vi "_GUID.vi"() -> (3 "uuid":string)   [LabVIEW 2014, in "TagDB(dev).lvlib"]
doc: "Generates a unique identification stringCopyright 2015 National Instruments Corporation\n\nLicensed under the Apache License, Version 2.0 (the \"License\"); you may not use this file except in compliance with the License. You may obtain a copy of the License at http://www.apache.org/licenses/LICENSE-2.0\nUnless required by applicable law or agreed to in writing, software distributed under the License is distributed on an \"AS IS\" BASIS, WITHOUT WARRANTIES OR CONDITIONS OF ANY KIND, either express or implied. See the License for the specific language governing permissions and limitations under the License."
uses:
  TagDB(dev).lvlib
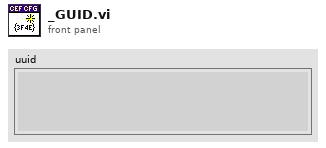
[diagram p1: front panel]
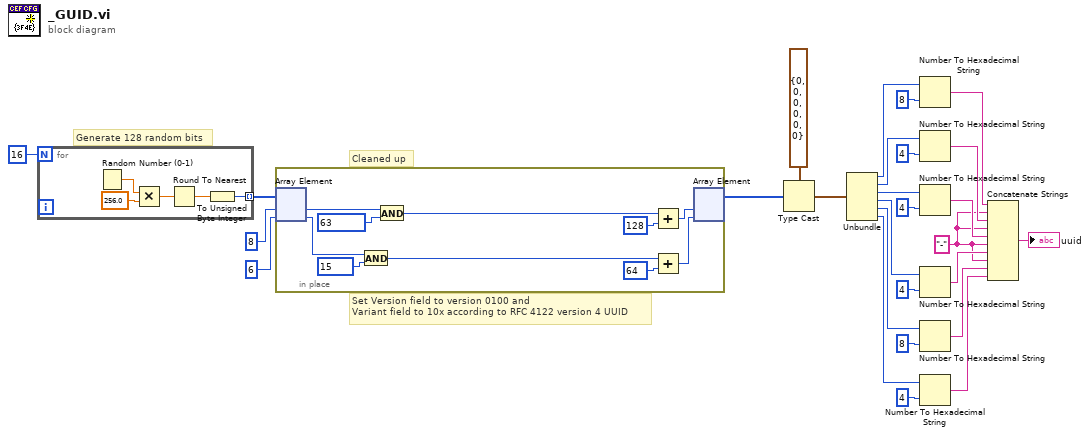
[diagram p0: block diagram]
diagram:
  w11 = "-" ("new element/subarray")
  # "Cleaned up"
  # "Set Version field to version 0100 and \nVariant field to 10x according to RFC 4122 version 4 UUID"
  # "Generate 128 random bits"
  n1 = for {
    N: 16 -> [_]
    tunnel: [w28] -> w26 mode=indexing
    n2 = Random Number (0-1)() -> (number: 0 to 1=w32:dbl)
    n3 = Multiply(x=w32, y=256.0) -> (x*y=w30:dbl)
    n4 = Round To Nearest(number=w30) -> (nearest integer value=w29:dbl)
    n5 = To Unsigned Byte Integer(number=w29) -> (unsigned 8bit integer=w28:u8)
  }
  n6 = in-place {
    n7 = in-place-array #1(w26, 8 ("index"), 6 ("index")) -> (w41:u8, w40:u8)
    n8 = And(x=w40, y=u8 15) -> (x .and. y?=w37:u8)
    n9 = And(x=w41, y=u8 63) -> (x .and. y?=w35:u8)
    n10 = Add(x=w35, y=u8 128) -> (x+y=w34:u8)
    n11 = Add(x=w37, y=u8 64) -> (x+y=w33:u8)
    n12 = in-place-array #1(w34, w33) -> (w2:u8[])  [unwired: 2 out]
  }
  n13 = Type Cast(type=cluster{u32, u16, u16, u16, u32, u16} {0, 0, 0, 0, 0, 0}, x=w2) -> (*(type *) &x=w22:cluster{u32, u16, u16, u16, u32, u16})
  n14 = Unbundle(w22) -> (w8:u32, w7:u16, w6:u16, w5:u16, w4:u32, w3:u16)
  n15 = Number To Hexadecimal String(1:i16 8 ("width (-)"), 2:w8) -> (0:w15:string)
  n16 = Number To Hexadecimal String(1:i16 4 ("width (-)"), 2:w7) -> (0:w14:string)
  n17 = Number To Hexadecimal String(1:i16 4 ("width (-)"), 2:w6) -> (0:w13:string)
  n18 = Number To Hexadecimal String(1:i16 4 ("width (-)"), 2:w5) -> (0:w12:string)
  n19 = Number To Hexadecimal String(1:i16 8 ("width (-)"), 2:w4) -> (0:w10:string)
  n20 = Number To Hexadecimal String(1:i16 4 ("width (-)"), 2:w3) -> (0:w9:string)
  n21 = Concatenate Strings(w15, w11, w14, w11, w13, w11, w12, w11, w10, w9) -> (→"uuid":string)
